vi "Write Poll(ms).vi"(8 "error in (no error)":errorcluster, 10 "Poll(ms)":u32, 11 "Instruments in":refnum<class "Instruments.lvclass">) -> (0 "error out":errorcluster, 3 "Instruments out":refnum<class "Instruments.lvclass">)   [LabVIEW 2023, in "Instruments.lvlib" / "Instruments.lvclass"]
uses:
  Library/Instruments.lvclass
  Library/Instruments.lvclass/Instruments.ctl
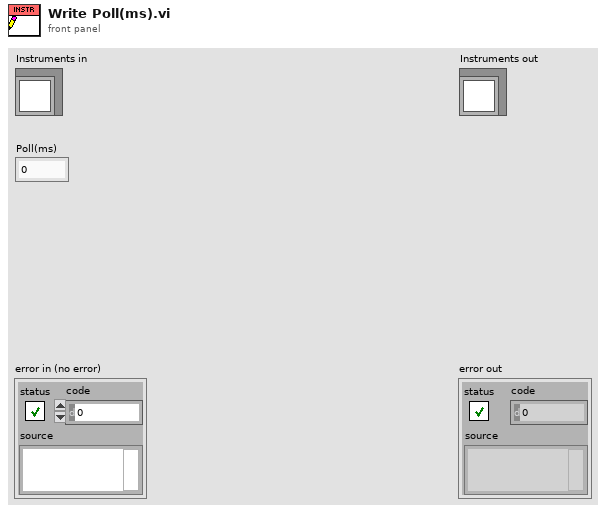
[diagram p1: front panel]
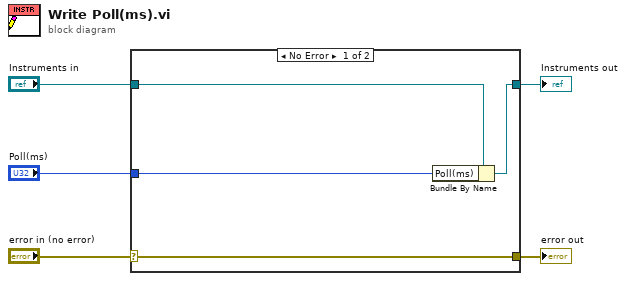
[diagram p0: block diagram]
diagram:
  n1 = case shown="No Error" "error in (no error)" {
    selector: "error in (no error)" -> [w9 w10]
    tunnel: [w9 w10] -> w4
    tunnel: [w7 w11] -> w2
    tunnel: "Instruments in" -> [w8 w11]
    tunnel: "Poll(ms)" -> [w6 _]
    frame No Error {
      n2 = Bundle By Name(cluster=w8, "Poll(ms)"=w6) -> (w7:refnum<class "Instruments.lvclass">)
    }
    frame Error {
    }
  }
  "error out" <- w4
  "Instruments out" <- w2
